vi "End.vi"(8 "error in (no error)":errorcluster, 11 "S4ACS_GUI in":refnum<class "S4GUI.lvclass">) -> (0 "error out":errorcluster, 3 "S4ACS_GUI out":refnum<class "S4GUI.lvclass">)   [LabVIEW 2018, in "S4GUI.lvclass"]
uses:
  S4GUI.lvclass
  S4GUI.lvclass/S4GUI.ctl
  Log/Log.lvclass
  Instrument/Instrument.lvclass
  GSserver/GSserver.lvclass
  Publisher/Publisher.lvclass
  WeatherStation/WeatherStation.lvclass
  TelFocus/TelFocus.lvclass
  TCS/TCS.lvclass
  Acquisition/Acquisition.lvclass
  SyncBox/Sync Box.lvclass
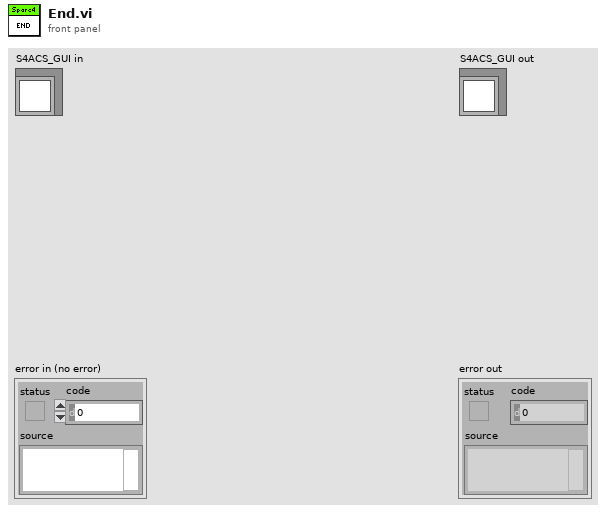
[diagram p1: front panel]
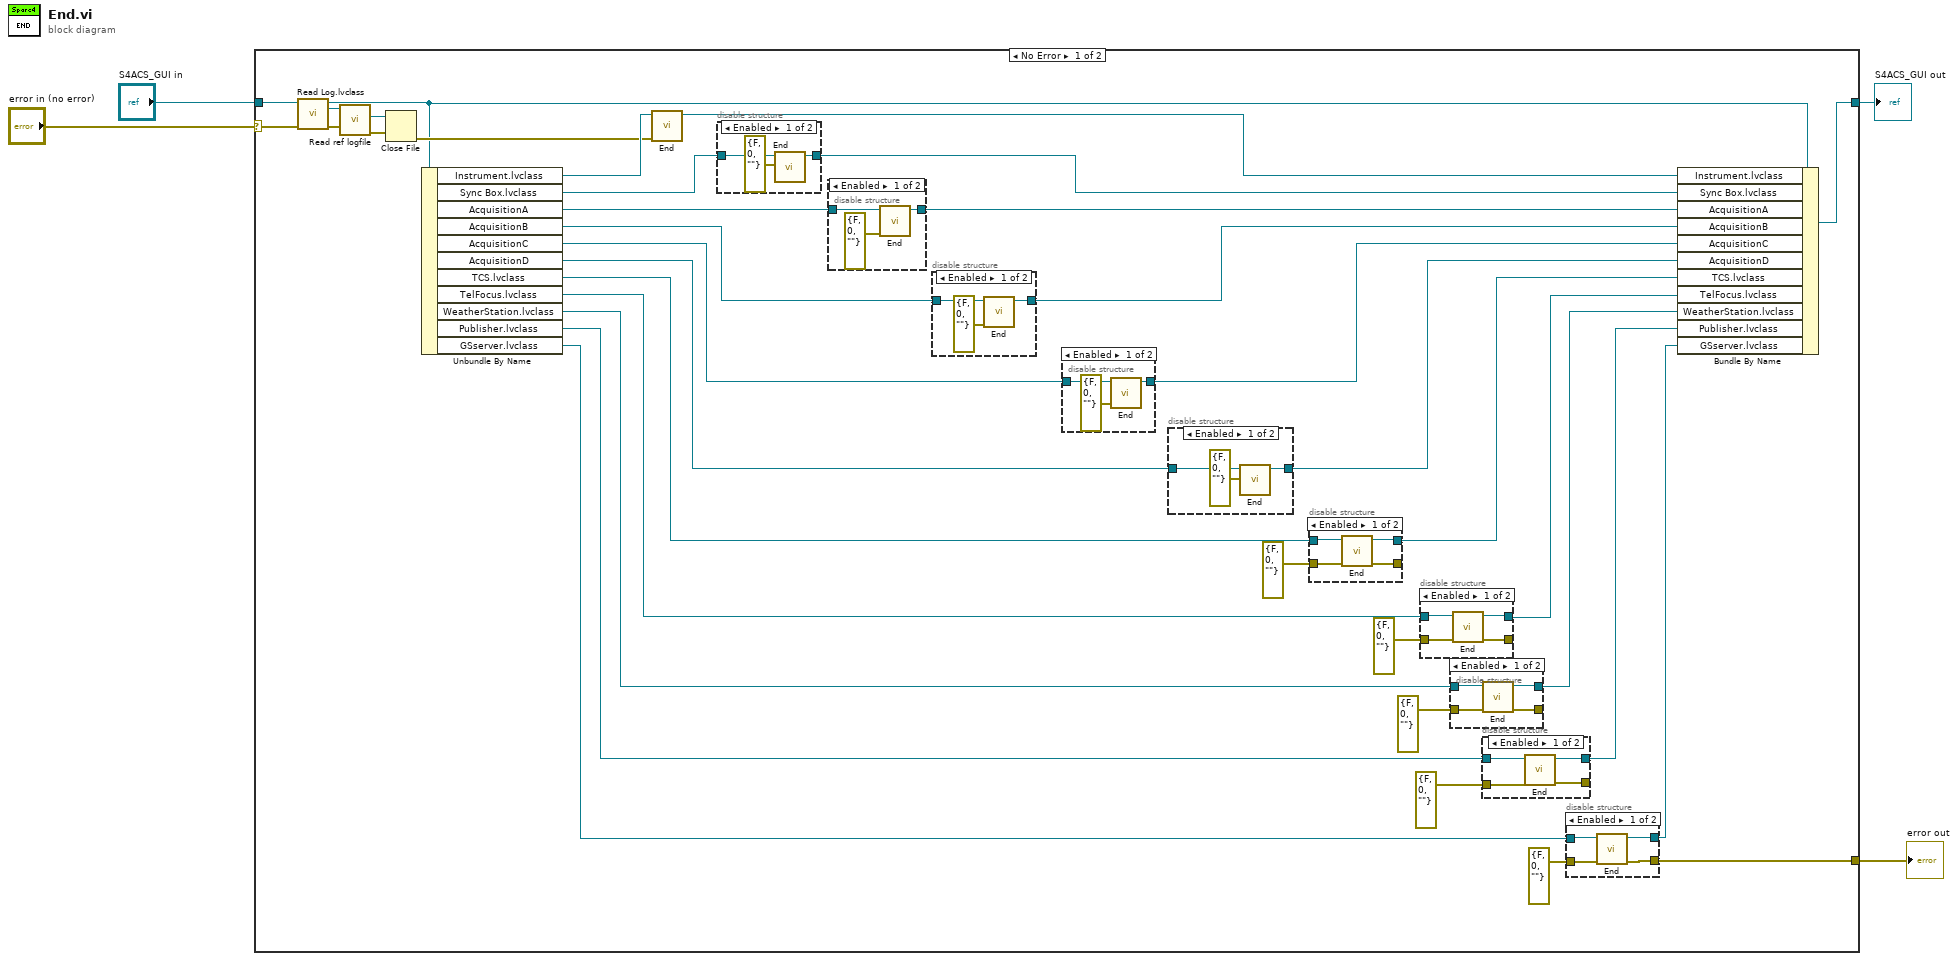
[diagram p0: block diagram]
diagram:
  n1 = case shown="No Error" "error in (no error)" {
    selector: "error in (no error)" -> [w23 w93]
    tunnel: [w5 w93] -> w3
    tunnel: [w38 w92] -> w1
    tunnel: "S4ACS_GUI in" -> [w24 w92]
    frame No Error {
      n2 = call-dynamic "Read Log.lvclass.vi"("error in (no error)"=w23, "S4GUI in"=w24) -> ("error out"=w20:errorcluster, "Log.lvclass"=w22:refnum<class "Log.lvclass">, "S4GUI out"=w18:refnum<class "S4GUI.lvclass">)  [unwired: 7 in]
      n3 = call-dynamic "Read ref logfile.vi"("error in (no error)"=w20, "Log in"=w22) -> ("error out"=w19:errorcluster, "ref logfile"=w21:refnum<file>)  [unwired: 7 in, 1 out]
      n4 = Close File(refnum=w21, error in=w19) -> (error out=w25:errorcluster)  [unwired: 1 out]
      n5 = Unbundle By Name(w18) -> ("Instrument.lvclass"=w30:refnum<class "Instrument.lvclass">, "Sync Box.lvclass"=w32:refnum<class "Sync Box.lvclass">, "AcquisitionA"=w41:refnum<class "Acquisition.lvclass">, "AcquisitionB"=w40:refnum<class "Acquisition.lvclass">, "AcquisitionC"=w37:refnum<class "Acquisition.lvclass">, "AcquisitionD"=w39:refnum<class "Acquisition.lvclass">, "TCS.lvclass"=w28:refnum<class "TCS.lvclass">, "TelFocus.lvclass"=w16:refnum<class "TelFocus.lvclass">, "WeatherStation.lvclass"=w13:refnum<class "WeatherStation.lvclass">, "Publisher.lvclass"=w11:refnum<class "Publisher.lvclass">, "GSserver.lvclass"=w7:refnum<class "GSserver.lvclass">)
      n6 = call-dynamic "End.vi"("error in (no error)"=w25, "Server in"=w30) -> ("Server out"=w29:refnum<class "Instrument.lvclass">)  [unwired: 8 in, 1 out]
      n7 = disable-structure shown="Enabled" {
        disable-tunnel: w32 -> [w90 w91]
        disable-tunnel: [w89 w91] -> w31
        frame Enabled {
          n8 = call-dynamic "End.vi"("error in (no error)"=errorcluster {"status"=FALSE, "code"=0, "source"=""}, "Server in"=w90) -> ("Server out"=w89:refnum<class "Sync Box.lvclass">)  [unwired: 8 in, 1 out]
        }
        frame Disabled {
        }
      }
      n9 = disable-structure shown="Enabled" {
        disable-tunnel: w41 -> [w76 w77]
        disable-tunnel: [w75 w77] -> w36
        frame Enabled {
          n10 = call-dynamic "End.vi"("error in (no error)"=errorcluster {"status"=FALSE, "code"=0, "source"=""}, "Acquisition in"=w76) -> ("Acquisition out"=w75:refnum<class "Acquisition.lvclass">)  [unwired: 8 in, 1 out]
        }
        frame Disabled {
        }
      }
      n11 = disable-structure shown="Enabled" {
        disable-tunnel: w40 -> [w86 w87]
        disable-tunnel: [w85 w87] -> w35
        frame Enabled {
          n12 = call-dynamic "End.vi"("error in (no error)"=errorcluster {"status"=FALSE, "code"=0, "source"=""}, "Acquisition in"=w86) -> ("Acquisition out"=w85:refnum<class "Acquisition.lvclass">)  [unwired: 8 in, 1 out]
        }
        frame Disabled {
        }
      }
      n13 = disable-structure shown="Enabled" {
        disable-tunnel: w37 -> [w72 w73]
        disable-tunnel: [w71 w73] -> w34
        frame Enabled {
          n14 = call-dynamic "End.vi"("error in (no error)"=errorcluster {"status"=FALSE, "code"=0, "source"=""}, "Acquisition in"=w72) -> ("Acquisition out"=w71:refnum<class "Acquisition.lvclass">)  [unwired: 8 in, 1 out]
        }
        frame Disabled {
        }
      }
      n15 = disable-structure shown="Enabled" {
        disable-tunnel: w39 -> [w68 w69]
        disable-tunnel: [w67 w69] -> w33
        frame Enabled {
          n16 = call-dynamic "End.vi"("error in (no error)"=errorcluster {"status"=FALSE, "code"=0, "source"=""}, "Acquisition in"=w68) -> ("Acquisition out"=w67:refnum<class "Acquisition.lvclass">)  [unwired: 8 in, 1 out]
        }
        frame Disabled {
        }
      }
      n17 = disable-structure shown="Enabled" {
        disable-tunnel: w28 -> [w81 w83]
        disable-tunnel: [w80 w83] -> w27
        disable-tunnel: [w79 w82] -> _
        disable-tunnel: errorcluster {"status"=FALSE, "code"=0, "source"=""} ("error in (no error)") -> [w78 w82]
        frame Enabled {
          n18 = call-dynamic "End.vi"("error in (no error)"=w78, "Server in"=w81) -> ("error out"=w79:errorcluster, "Server out"=w80:refnum<class "TCS.lvclass">)  [unwired: 8 in]
        }
        frame Disabled {
        }
      }
      n19 = disable-structure shown="Enabled" {
        disable-tunnel: w16 -> [w63 w65]
        disable-tunnel: [w62 w65] -> w15
        disable-tunnel: [w61 w64] -> _
        disable-tunnel: errorcluster {"status"=FALSE, "code"=0, "source"=""} ("error in (no error)") -> [w60 w64]
        frame Enabled {
          n20 = call-dynamic "End.vi"("error in (no error)"=w60, "TelFocus in"=w63) -> ("error out"=w61:errorcluster, "TelFocus out"=w62:refnum<class "TelFocus.lvclass">)  [unwired: 8 in]
        }
        frame Disabled {
        }
      }
      n21 = disable-structure shown="Enabled" {
        disable-tunnel: w13 -> [w57 w59]
        disable-tunnel: [w56 w59] -> w12
        disable-tunnel: [w55 w58] -> _
        disable-tunnel: errorcluster {"status"=FALSE, "code"=0, "source"=""} ("error in (no error)") -> [w54 w58]
        frame Enabled {
          n22 = call-dynamic "End.vi"("error in (no error)"=w54, "WeatherStation in"=w57) -> ("error out"=w55:errorcluster, "WeatherStation out"=w56:refnum<class "WeatherStation.lvclass">)  [unwired: 8 in]
        }
        frame Disabled {
        }
      }
      n23 = disable-structure shown="Enabled" {
        disable-tunnel: w11 -> [w51 w52]
        disable-tunnel: errorcluster {"status"=FALSE, "code"=0, "source"=""} ("error in (no error)") -> [w50 w53]
        disable-tunnel: [w49 w53] -> _
        disable-tunnel: [w48 w52] -> w9
        frame Enabled {
          n24 = call-dynamic "End.vi"("error in (no error)"=w50, "Client in"=w51) -> ("error out"=w49:errorcluster, "Client out"=w48:refnum<class "Publisher.lvclass">)  [unwired: 8 in]
        }
        frame Disabled {
        }
      }
      n25 = disable-structure shown="Enabled" {
        disable-tunnel: w7 -> [w45 w47]
        disable-tunnel: [w44 w47] -> w6
        disable-tunnel: [w43 w46] -> w5
        disable-tunnel: errorcluster {"status"=FALSE, "code"=0, "source"=""} ("error in (no error)") -> [w42 w46]
        frame Enabled {
          n26 = call-dynamic "End.vi"("error in (no error)"=w42, "Server in"=w45) -> ("error out"=w43:errorcluster, "Server out"=w44:refnum<class "GSserver.lvclass">)  [unwired: 8 in]
        }
        frame Disabled {
        }
      }
      n27 = Bundle By Name(cluster=w18, "Instrument.lvclass"=w29, "Sync Box.lvclass"=w31, "AcquisitionA"=w36, "AcquisitionB"=w35, "AcquisitionC"=w34, "AcquisitionD"=w33, "TCS.lvclass"=w27, "TelFocus.lvclass"=w15, "WeatherStation.lvclass"=w12, "Publisher.lvclass"=w9, "GSserver.lvclass"=w6) -> (w38:refnum<class "S4GUI.lvclass">)
    }
    frame Error {
    }
  }
  "error out" <- w3
  "S4ACS_GUI out" <- w1
